vi "CanakitRelays.vi"(6 "Write String":string="*IDN?\r\n", 8 "Error In":errorcluster, 9 "Set Relays":cluster{"1":bool, "2":bool, "3":bool, "4":bool}, 10 "Function":T1(ring), 11 "VISA resource name":refnum<visa-resource-name>="COM1") -> (0 "Error Out":errorcluster, 1 "Get Relays":cluster{"1":bool, "2":bool, "3":bool, "4":bool}, 2 "Read String":string)   [LabVIEW 2014]
uses:
  <vilib>/Instr/_visa.llb/VISA Configure Serial Port (Instr).vi
panel:
  # "LICENSED MATERIALS – PROPERTY OF IBM\nCopyright IBM Corp. 2016,\nALL RIGHTS RESERVED"
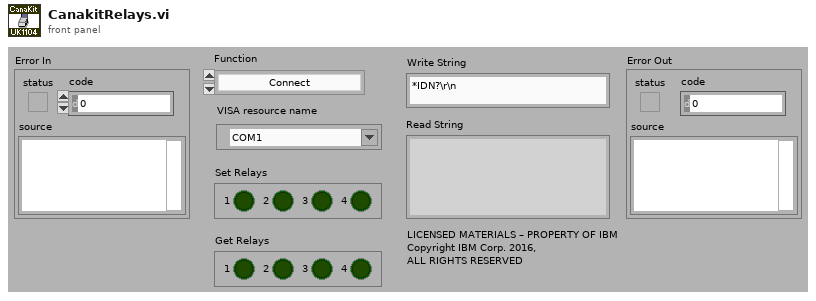
[diagram p1: front panel]
types:
  T1 = enum16{"Connect", "Generic I/O", "Initialize", "Get Configuration", "Switch Relay", "Info", "Disconnect"}
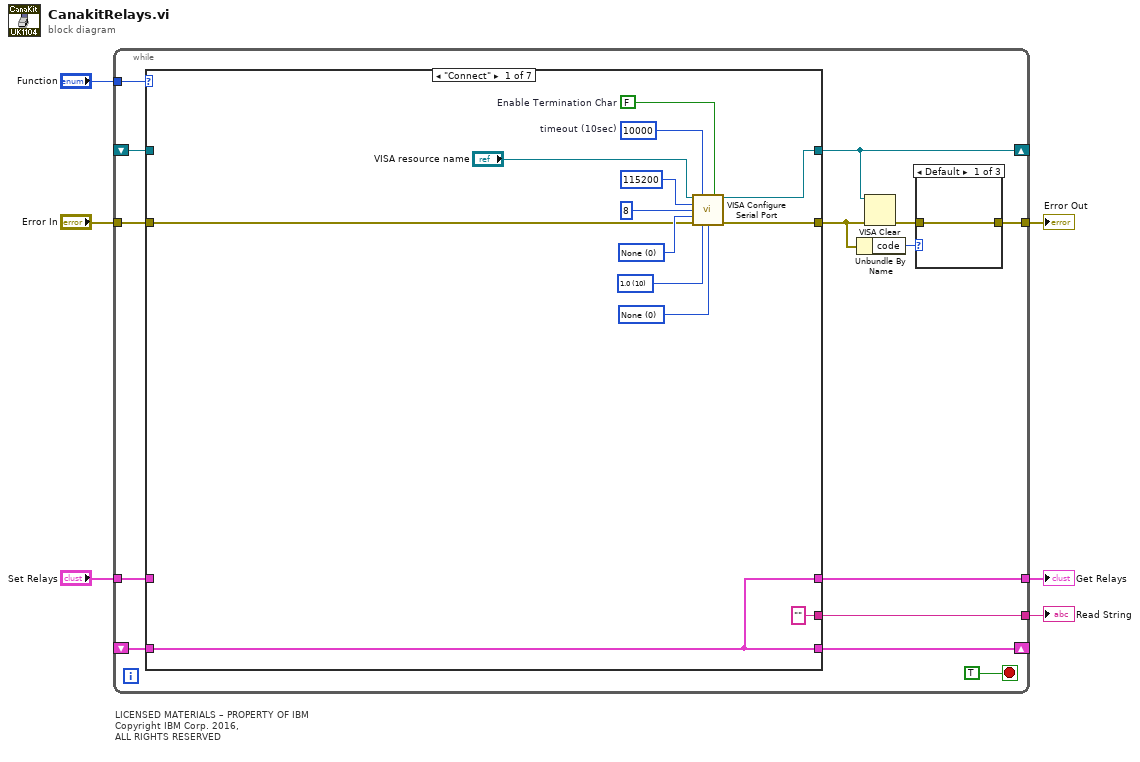
[diagram p0: block diagram]
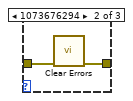
[diagram p2: hidden frame]
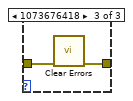
[diagram p3: hidden frame]
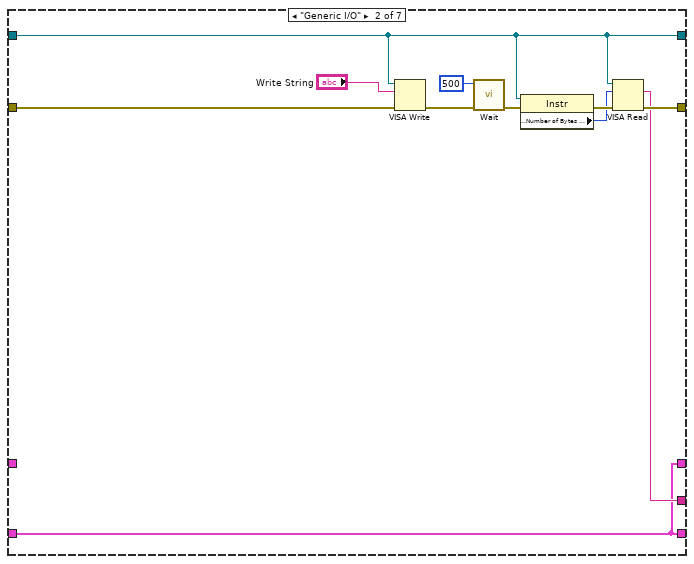
[diagram p4: hidden frame]
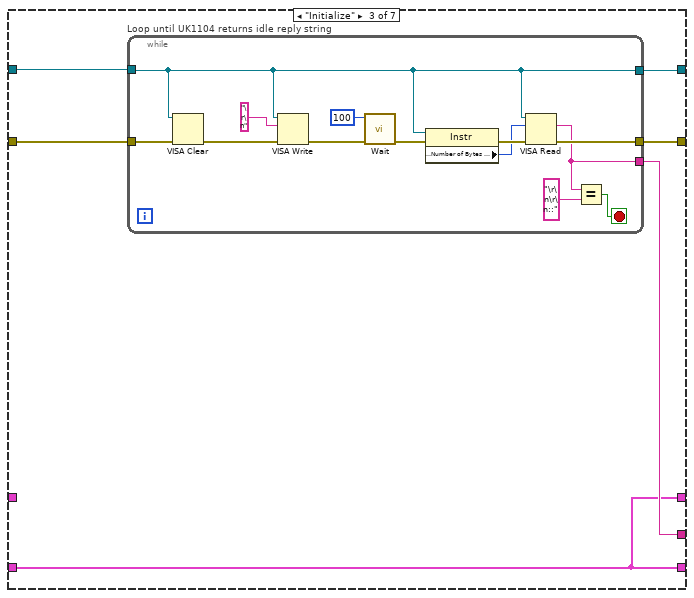
[diagram p5: hidden frame]
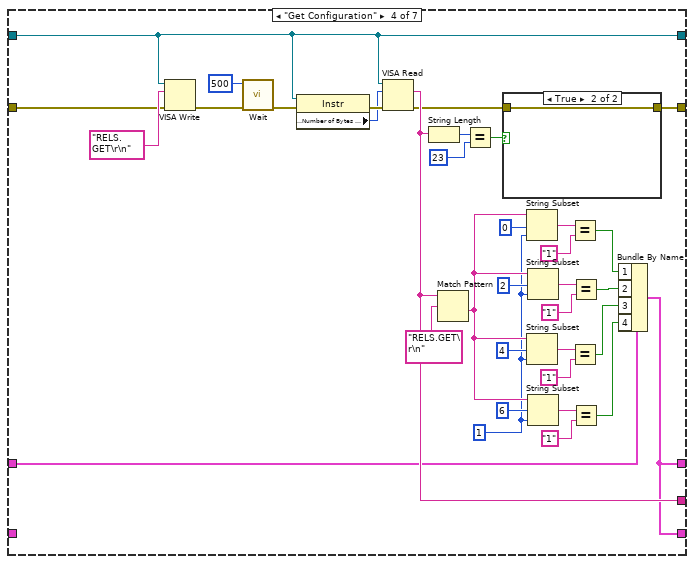
[diagram p6: hidden frame]
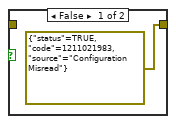
[diagram p7: hidden frame]
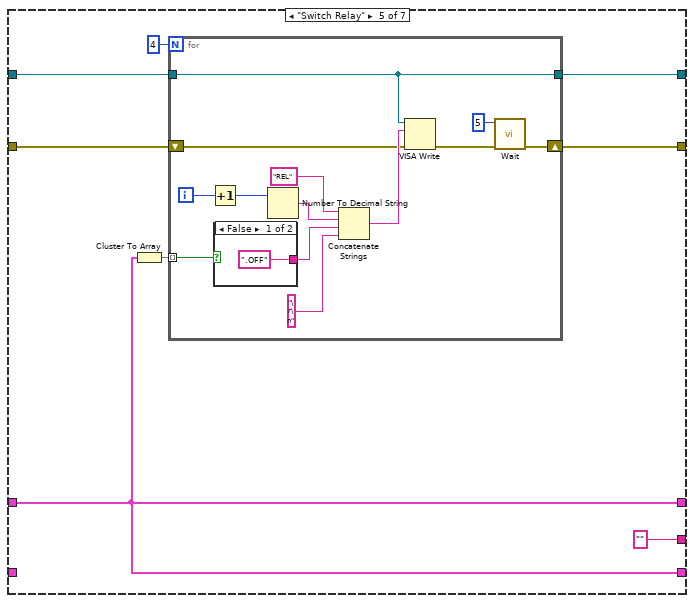
[diagram p8: hidden frame]
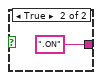
[diagram p9: hidden frame]
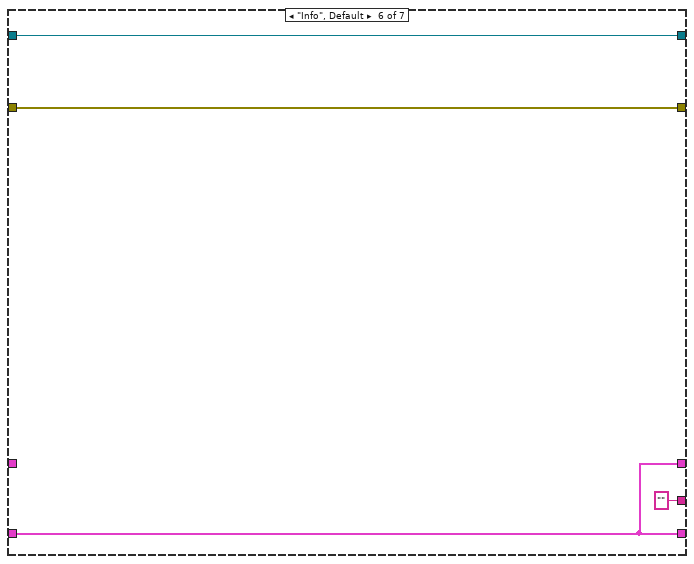
[diagram p10: hidden frame]
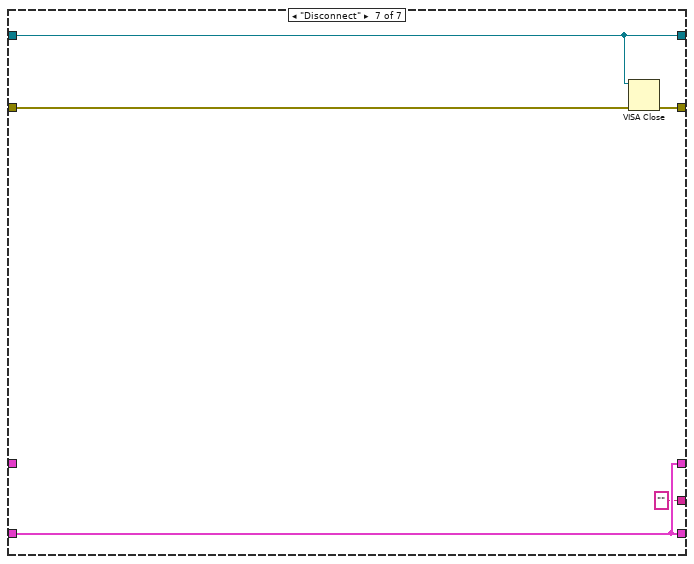
[diagram p11: hidden frame]
diagram:
  # "LICENSED MATERIALS – PROPERTY OF IBM\nCopyright IBM Corp. 2016,\nALL RIGHTS RESERVED"
  n1 = while {
    tunnel: "Function" -> [w20]
    tunnel: [w11] -> w5
    tunnel: "Error In" -> [w13]
    tunnel: "Set Relays" -> [w19]
    tunnel: [w18] -> w2
    shift-right: [w15] -> _
    shift-left: _ -> [w14]
    tunnel: [w16] -> w1
    shift-right: [w7] -> _
    shift-left: _ -> [w12]
    stop <- TRUE stop-if-true
    n2 = case shown="\"Connect\"" w20 {
      tunnel: [w28 w39 w54 w70 w111 w132 w135] -> w7
      tunnel: [w29 w49 w53 w102 w109 w131 w137] -> w9
      tunnel: w12 -> [_ w39 w55 w70 w110 w132 w135]
      tunnel: w19 -> [_ _ _ w100 w107 _ _]
      tunnel: ["" ("read buffer") w48 w52 w101 "" ("read buffer") "" ("read buffer") "" ("read buffer")] -> w18
      tunnel: [w27 w47 w51 w99 w107 w130 w134] -> w15
      tunnel: [w27 w47 w51 w99 w107 w130 w134] -> w16
      tunnel: w14 -> [w27 w47 w51 _ _ w130 w134]
      tunnel: w13 -> [w30 w45 w50 w69 w106 w131 w136]
      frame "Connect" {
        w37 = u16 0 items=["None"=0, "XON/XOFF"=1, "RTS/CTS"=2, "DTR/DSR"=4] ("flow control")
        w36 = u16 10 items=["1.0"=10, "1.5"=15, "2.0"=20] ("stop bits")
        w33 = u16 0 items=["None", "Odd", "Even", "Mark", "Space"] ("parity")
        w34 = u32 10000  # timeout (10sec)
        w35 = FALSE  # Enable Termination Char
        n3 = call-poly "VISA Configure Serial Port"("VISA resource name"="VISA resource name", "timeout (10sec)"=w34, "Enable Termination\nChar (T)"=w35, "baud rate (9600)"=u32 115200 ("baud rate"), "data bits (8)"=u16 8 ("data bits"), "parity (0:none)"=w33, "error in (no error)"=w30, "stop bits (10: 1 bit)"=w36, "flow control (0:none)"=w37) -> ("VISA resource name out"=w28:refnum<visa-resource-name>, "error out"=w29:errorcluster)  [unwired: 5 out]
      }
      frame "Generic I/O" {
        n4 = VISA Write(VISA resource name=w39, write buffer="Write String", error in (no error)=w45) -> (error out=w44:errorcluster)  [unwired: 2 out]
        n5 = call "Wait.vi"("error in (no error)"=w44, "milliseconds to wait"=u32 500 ("delay before read (ms)")) -> ("error out"=w43:errorcluster)  [unwired: 9 in]
        n6 = property class="Instr"(reference=w39, error in=w43) -> (error out=w41:errorcluster, "Serial Settings:Number of Bytes at Serial Port"=w40:u32)  [unwired: 1 out]
        n7 = VISA Read(VISA resource name=w39, byte count=w40, error in (no error)=w41) -> (read buffer=w48:string, error out=w49:errorcluster)  [unwired: 2 out]
      }
      frame "Initialize" {
        n8 = while "Loop until UK1104 returns idle reply string" {
          tunnel: w55 -> [w56]
          tunnel: [w56] -> w54
          tunnel: [w65] -> w53
          tunnel: [w64] -> w52
          tunnel: w50 -> [w63]
          stop <- w66 stop-if-true
          n9 = VISA Clear(VISA resource name=w56, error in (no error)=w63) -> (error out=w57:errorcluster)  [unwired: 1 out]
          n10 = VISA Write(VISA resource name=w56, write buffer="\r\n" ("string to write 2"), error in (no error)=w57) -> (error out=w68:errorcluster)  [unwired: 2 out]
          n11 = call "Wait.vi"("error in (no error)"=w68, "milliseconds to wait"=u32 100 ("delay before read (ms)")) -> ("error out"=w67:errorcluster)  [unwired: 9 in]
          n12 = property class="Instr"(reference=w56, error in=w67) -> (error out=w61:errorcluster, "Serial Settings:Number of Bytes at Serial Port"=w60:u32)  [unwired: 1 out]
          n13 = VISA Read(VISA resource name=w56, byte count=w60, error in (no error)=w61) -> (read buffer=w64:string, error out=w65:errorcluster)  [unwired: 2 out]
          n14 = Equal?(x=w64, y="\r\n\r\n::" ("string to write 2")) -> (x = y?=w66:bool)
        }
      }
      frame "Get Configuration" {
        w76 = 1 ("length (rest)")
        n15 = VISA Write(VISA resource name=w70, write buffer="RELS.GET\r\n" ("string to write 2"), error in (no error)=w69) -> (error out=w103:errorcluster)  [unwired: 2 out]
        n16 = call "Wait.vi"("error in (no error)"=w103, "milliseconds to wait"=u32 500 ("delay before read (ms)")) -> ("error out"=w98:errorcluster)  [unwired: 9 in]
        n17 = property class="Instr"(reference=w70, error in=w98) -> (error out=w95:errorcluster, "Serial Settings:Number of Bytes at Serial Port"=w79:u32)  [unwired: 1 out]
        n18 = VISA Read(VISA resource name=w70, byte count=w79, error in (no error)=w95) -> (read buffer=w101:string, error out=w71:errorcluster)  [unwired: 2 out]
        n19 = String Length(string=w101) -> (length=w74:i32)
        n20 = Match Pattern(string=w101, regular expression="RELS.GET\r\n" ("read string")) -> (after substring=w77:string)  [unwired: 4 out]
        n21 = Equal?(x=w74, y=23) -> (x = y?=w72:bool)
        n22 = case shown="True" w72 {
          tunnel: w71 -> [_ w105]
          tunnel: [errorcluster {"status"=TRUE, "code"=1211021983, "source"="Configuration Misread"} ("Error Out 2") w105] -> w102
          frame False {
          }
          frame True {
          }
        }
        n23 = String Subset(string=w77, offset (0)=0 ("length (rest)"), length (rest)=w76) -> (substring=w75:string)
        n24 = String Subset(string=w77, offset (0)=4 ("length (rest)"), length (rest)=w76) -> (substring=w84:string)
        n25 = String Subset(string=w77, offset (0)=2 ("length (rest)"), length (rest)=w76) -> (substring=w83:string)
        n26 = String Subset(string=w77, offset (0)=6 ("length (rest)"), length (rest)=w76) -> (substring=w87:string)
        n27 = Equal?(x=w75, y="1" ("read string")) -> (x = y?=w91:bool)
        n28 = Equal?(x=w84, y="1" ("read string")) -> (x = y?=w93:bool)
        n29 = Equal?(x=w83, y="1" ("read string")) -> (x = y?=w92:bool)
        n30 = Equal?(x=w87, y="1" ("read string")) -> (x = y?=w94:bool)
        n31 = Bundle By Name(cluster=w100, "1"=w91, "2"=w92, "3"=w93, "4"=w94) -> (w99:cluster{"1":bool, "2":bool, "3":bool, "4":bool})
      }
      frame "Switch Relay" {
        n32 = Cluster To Array(cluster=w107) -> (array=w113:bool[])
        n33 = for {
          N: 4 -> [_]
          tunnel: w113 -> [w123] mode=indexing
          shift-right: [w116] -> w109
          shift-left: w106 -> [w114]
          tunnel: w110 -> [w115]
          tunnel: [w115] -> w111
          i -> [w119]
          n34 = Increment(x=w119) -> (x+1=w118:i32)
          n35 = case shown="False" w123 {
            tunnel: [".OFF" ("string to write 2") ".ON" ("string to write 2")] -> w122
            frame False {
            }
            frame True {
            }
          }
          n36 = Number To Decimal String(number=w118) -> (decimal integer string=w125:string)  [unwired: 1 out]
          n37 = Concatenate Strings("REL" ("string to write 2"), w125, w122, "\r\n" ("string to write 2")) -> (w121:string)
          n38 = VISA Write(VISA resource name=w115, write buffer=w121, error in (no error)=w114) -> (error out=w120:errorcluster)  [unwired: 2 out]
          n39 = call "Wait.vi"("error in (no error)"=w120, "milliseconds to wait"=u32 5 ("delay before read (ms)")) -> ("error out"=w116:errorcluster)  [unwired: 9 in]
        }
      }
      frame "Info", Default {
      }
      frame "Disconnect" {
        n40 = VISA Close(VISA resource name=w135, error in (no error)=w136) -> (error out=w137:errorcluster)
      }
    }
    n41 = Unbundle By Name(w9) -> ("code"=w10:i32)
    n42 = VISA Clear(VISA resource name=w7, error in (no error)=w9) -> (error out=w8:errorcluster)  [unwired: 1 out]
    n43 = case shown="Default" w10 {
      tunnel: [w21 w23 w25] -> w11
      tunnel: w8 -> [w21 w22 w24]
      frame Default {
      }
      frame 1073676294 {
        n44 = call <vilib>:"Clear Errors.vi"("error in (no error)"=w22) -> ("error out"=w23:errorcluster)  [unwired: 5 in, 1 out]
      }
      frame 1073676418 {
        n45 = call <vilib>:"Clear Errors.vi"("error in (no error)"=w24) -> ("error out"=w25:errorcluster)  [unwired: 5 in, 1 out]
      }
    }
  }
  "Error Out" <- w5
  "Read String" <- w2
  "Get Relays" <- w1
